vi "Waveplate control panel.vi"(4 "PC WP angle":dbl, 5 "Left or right?":dbl(ring)=80.7 items=["Equal"=58.2, "Right"=35.7, "Left"=80.7], 6 "Pump WP angle":dbl, 7 "Waveplate or Pockels cell?":dbl(ring)=55.98 items=["Waveplate"=71.5, "Pockels cell"=26.5], 8 "L/R WP angle":dbl, 9 "Manual?":bool, 10 "Move waveplates":bool, 11 "Home Button":bool) -> (2 "VISA handle out":refnum<visa-resource-name>, 3 "Final positions":dbl[](array[numeric]))   [LabVIEW 2013]
doc: "Demonstrates the fundamentals of the State Machine design pattern in LabVIEW. A state machine, in its simplest form, is a case structure within a while loop, with a state enum wired to a shift register on the loop to define the execution of different cases (or \"states\") of the case structure on different iterations of the loop."
uses:
  Source/State Machine Fundamentals - State Enum.ctl
panel:
  in  "Axis 3\n(Pump)":bool=TRUE
  in  "Axis 2\n(WP/PC)":bool=TRUE
  in  "Axis 1\n(L/R)":bool=TRUE
  in  "Serial port":u8=3
  out "Moving":bool
  out "Initializing":bool
  out "Error out":errorcluster
  out "Moving axis":i32
  in  "Error in":errorcluster
  in  "Stop":bool
  # "Instructions: Start VI. All three SMC100 motion controllers will automatically initialize; this will\ntake several seconds for each and requires homing the stages. Choose waveplate/Pockels cell\nand left/right, OR turn on Manual and set desired angles for each stage. The pump waveplate\nalways uses its manual value. Press Move Waveplates to initiate motion. If any stage gives a \n\"Controller is not in the ready state\" error, it may be necessary to re-initialize by pressing Initialize."
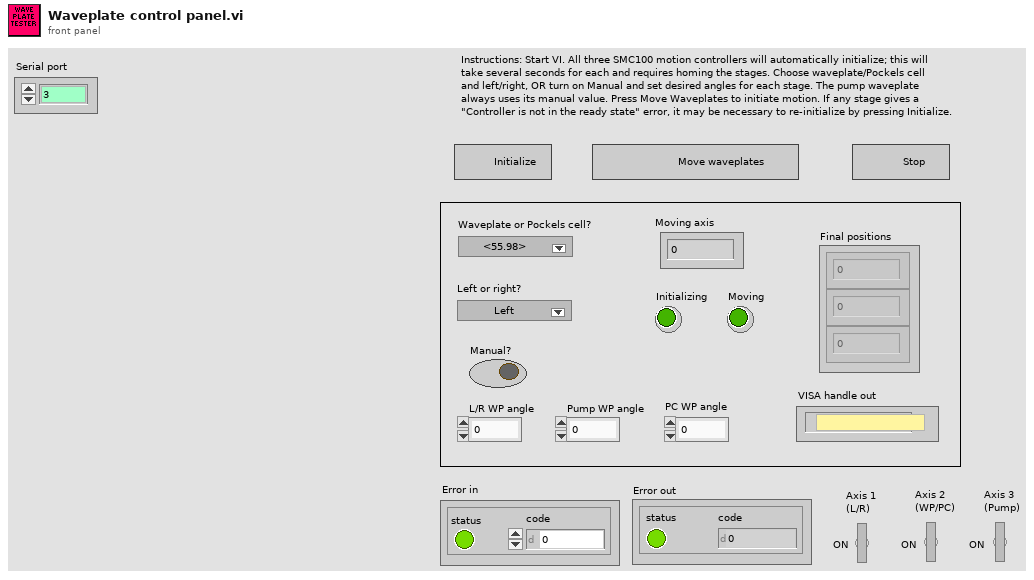
[diagram p1: front panel]
types:
  T1 = typedef "State Machine Fundamentals - State Enum.ctl" = enum16{"Initialize", "Wait for go", "Move", "Stop"}
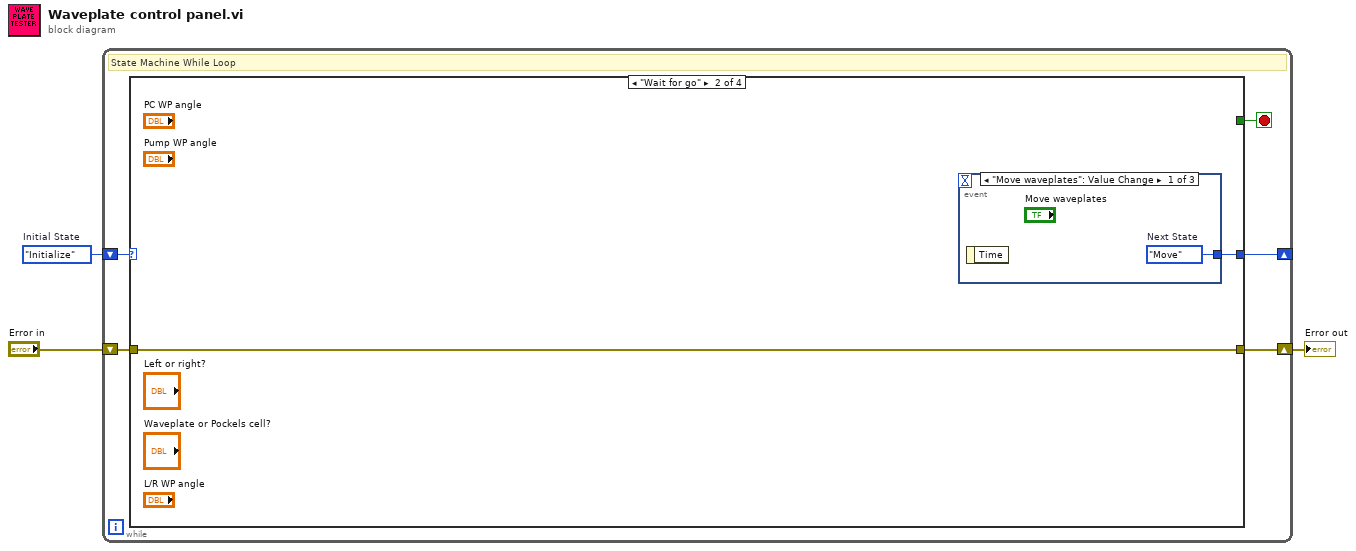
[diagram p0: block diagram]
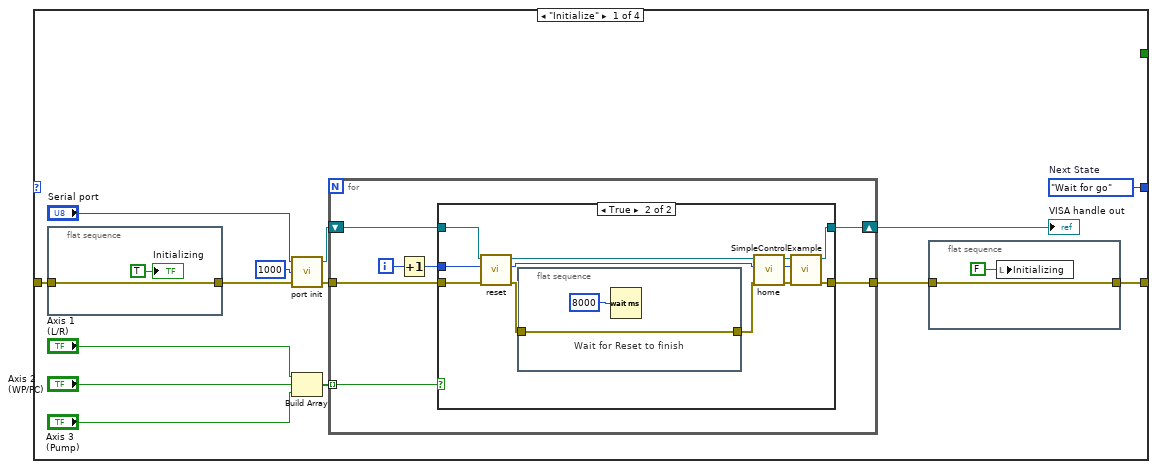
[diagram p2: hidden frame]
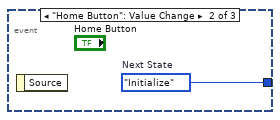
[diagram p4: hidden frame]
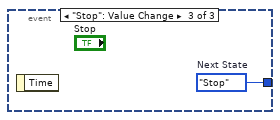
[diagram p5: hidden frame]
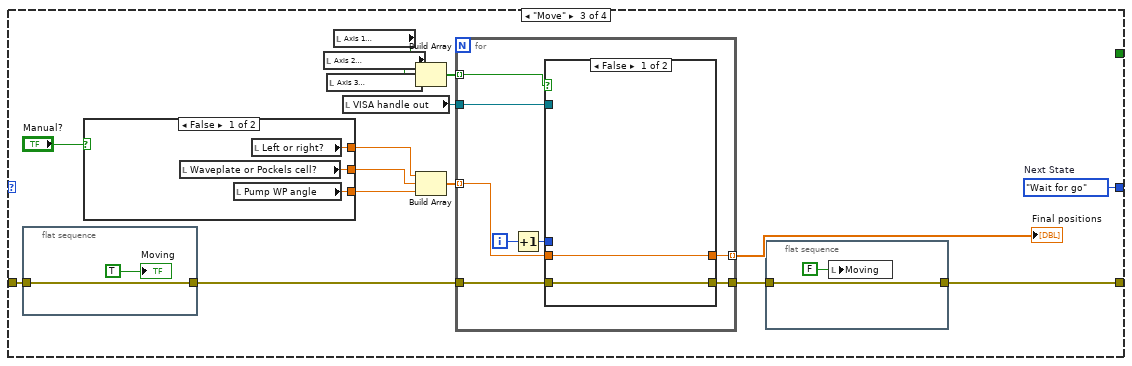
[diagram p6: hidden frame]
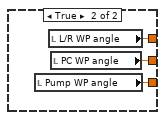
[diagram p7: hidden frame]
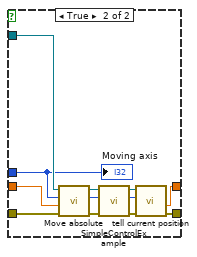
[diagram p8: hidden frame]
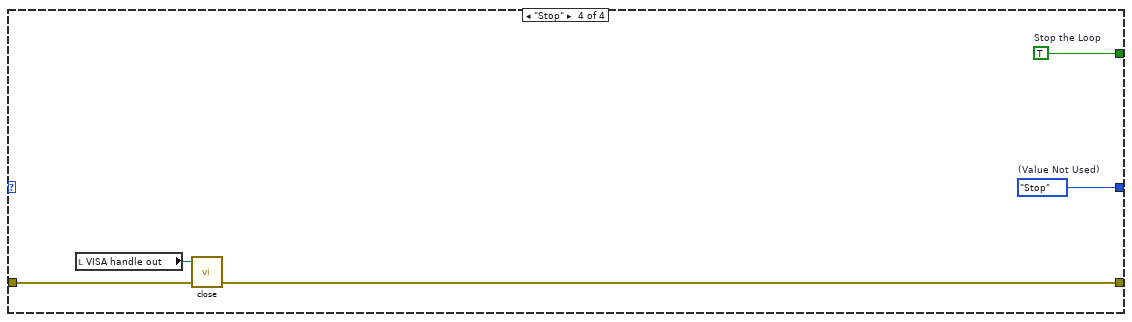
[diagram p9: hidden frame]
diagram:
  w3 = State_Machine_Fundamentals_-_State_Enum."Initialize"  # Initial State
  n1 = while {
    shift-right: [w7] -> _
    shift-left: w3 -> [w8]
    shift-right: [w4] -> w1
    shift-left: "Error in" -> [w5]
    stop <- w6 stop-if-true
    # "State Machine While Loop"
    n2 = case "State Machine Case Structure" shown="\"Wait for go\"" w8 {
      tunnel: [w22 w51 w69 w107] -> w7
      tunnel: [_ _ _ w106] -> w6
      tunnel: w5 -> [w21 w50 w64 w105]
      tunnel: [w20 w50 w61 w104] -> w4
      frame "Initialize" {
        w22 = State_Machine_Fundamentals_-_State_Enum."Wait for go"  # Next State
        n3 = flat-sequence {
          tunnel: w21 -> [w49]
          tunnel: [w49] -> w15
          frame #0 {
            "Initializing" <- TRUE ("Initializing")
          }
        }
        n4 = call "port init.vi"("error in"=w15, "Timeout (ms)"=u32 1000 ("Timeout (300 ms)"), "SerialPort"="Serial port") -> ("error out"=w14:errorcluster, "Visa Handle"=w16:refnum<visa-resource-name>)  [unwired: 1 in]
        n5 = Build Array("Axis 1\n(L/R)", "Axis 2\n(WP/PC)", "Axis 3\n(Pump)") -> (w9:bool[])
        n6 = for {
          tunnel: w14 -> [w27]
          shift-right: [w29] -> w19
          shift-left: w16 -> [w28]
          tunnel: [w26] -> w13
          tunnel: w9 -> [w23] mode=indexing
          i -> [w25]
          n7 = Increment(x=w25) -> (x+1=w24:i32)
          n8 = case shown="True" w23 {
            tunnel: [w31 w36] -> w29
            tunnel: w28 -> [w31 w35]
            tunnel: w27 -> [w30 w34]
            tunnel: [w30 w33] -> w26
            tunnel: w24 -> [_ w32]
            frame False {
            }
            frame True {
              n9 = call "reset.vi"("error in"=w34, "Axis in"=w32, "VISA Handle in"=w35) -> ("error out"=w39:errorcluster, "Axis out"=w40:i32, "VISA Handle out"=w37:refnum<visa-resource-name>)  [unwired: 3 in, 1 out]
              n10 = flat-sequence {
                tunnel: [w44] -> w38
                tunnel: w39 -> [w44]
                frame #0 {
                  # "Wait for Reset to finish"
                  n11 = Wait (ms)(milliseconds to wait=u32 8000) -> ()  [unwired: 1 out]
                }
              }
              n12 = call "home.vi"("error in"=w38, "Axis in"=w40, "VISA Handle in"=w37) -> ("error out"=w42:errorcluster, "Axis out"=w41:i32, "VISA Handle out"=w43:refnum<visa-resource-name>)  [unwired: 3 in, 1 out]
              n13 = call "SimpleControlExample.vi"("error in"=w42, "Axis in"=w41, "VISA Handle in"=w43) -> ("error out"=w33:errorcluster, "VISA Handle out"=w36:refnum<visa-resource-name>)  [unwired: 2 in, 3 out]
            }
          }
        }
        "VISA handle out" <- w19
        n14 = flat-sequence {
          tunnel: w13 -> [w47]
          tunnel: [w47] -> w20
          frame #0 {
            n15 = local write "Initializing"(FALSE ("Initializing")) -> ()
          }
        }
      }
      frame "Wait for go" {
        # "Wait for Event - An Event Structure is used to monitor the user interface for events. In each frame of the Event Structure, the next state of the state machine is specified based on which button was pressed."
        n16 = event shown="[0] \"Move waveplates\": Value Change" {
          selector: _ -> [_ _ _]
          dyn-events: _ -> [_ _ _]
          timeout: _ -> [_ _ _]
          tunnel: [w52 w53 w54] -> w51
          event "Move waveplates": Value Change {
            w52 = State_Machine_Fundamentals_-_State_Enum."Move"  # Next State
            n17 = event-data() -> ()  [unwired: 1 in, 1 out]
          }
          event "Home Button": Value Change {
            w53 = State_Machine_Fundamentals_-_State_Enum."Initialize"  # Next State
            n18 = event-data() -> ()  [unwired: 1 in, 1 out]
          }
          event "Stop": Value Change {
            w54 = State_Machine_Fundamentals_-_State_Enum."Stop"  # Next State
            n19 = event-data() -> ()  [unwired: 1 in, 1 out]
          }
        }
      }
      frame "Move" {
        w69 = State_Machine_Fundamentals_-_State_Enum."Wait for go"  # Next State
        # "State 1 - Display a dialog box with a message specific to State 1, then go back to the Wait for Event state."
        n20 = flat-sequence {
          tunnel: w64 -> [w80]
          tunnel: [w80] -> w63
          frame #0 {
            "Moving" <- TRUE ("Moving")
          }
        }
        n21 = case shown="False" "Manual?" {
          tunnel: [w73 w76] -> w67
          tunnel: [w72 w75] -> w66
          tunnel: [w71 w74] -> w59
          frame False {
            n22 = local read "Waveplate or Pockels cell?"() -> (w72:dbl)
            n23 = local read "Pump WP angle"() -> (w71:dbl)
            n24 = local read "Left or right?"() -> (w73:dbl)
          }
          frame True {
            n25 = local read "Pump WP angle"() -> (w74:dbl)
            n26 = local read "L/R WP angle"() -> (w76:dbl)
            n27 = local read "PC WP angle"() -> (w75:dbl)
          }
        }
        n28 = local read "Axis 2\n(WP/PC)"() -> (w57:bool)
        n29 = local read "Axis 3\n(Pump)"() -> (w56:bool)
        n30 = local read "Axis 1\n(L/R)"() -> (w58:bool)
        n31 = local read "VISA handle out"() -> (w65:refnum<visa-resource-name>)
        n32 = Build Array(w58, w57, w56) -> (w55:bool[])
        n33 = Build Array(w67, w66, w59) -> (w68:dbl[])
        n34 = for {
          tunnel: [w88] -> w70 mode=indexing
          tunnel: w63 -> [w87]
          tunnel: [w86] -> w62
          tunnel: w68 -> [w85] mode=indexing
          tunnel: w65 -> [w84]
          tunnel: w55 -> [w83] mode=indexing
          i -> [w82]
          n35 = Increment(x=w82) -> (x+1=w81:i32)
          n36 = case shown="False" w83 {
            tunnel: [w89 w102] -> w88
            tunnel: w87 -> [w90 w101]
            tunnel: [w90 w100] -> w86
            tunnel: w85 -> [w89 w99]
            tunnel: w84 -> [_ w98]
            tunnel: w81 -> [_ w91]
            frame False {
            }
            frame True {
              n37 = call "Move absolute.vi"("error in"=w101, "New target position (units)"=w99, "Axis in"=w91, "VISA Handle in"=w98) -> ("error out"=w92:errorcluster, "Axis out"=w93:i32, "VISA Handle out"=w94:refnum<visa-resource-name>)  [unwired: 2 in, 1 out]
              n38 = call "SimpleControlExample.vi"("error in"=w92, "Axis in"=w93, "VISA Handle in"=w94) -> ("error out"=w95:errorcluster, "Axis out"=w96:i32, "VISA Handle out"=w97:refnum<visa-resource-name>)  [unwired: 2 in, 2 out]
              n39 = call "tell current position.vi"("error in"=w95, "Axis in"=w96, "VISA Handle in"=w97) -> ("error out"=w100:errorcluster, "Current position (units)"=w102:dbl)  [unwired: 2 in, 3 out]
              "Moving axis" <- w91
            }
          }
        }
        "Final positions" <- w70
        n40 = flat-sequence {
          tunnel: w62 -> [w77]
          tunnel: [w77] -> w61
          frame #0 {
            n41 = local write "Moving"(FALSE ("Moving")) -> ()
          }
        }
      }
      frame "Stop" {
        w106 = TRUE  # Stop the Loop
        w107 = State_Machine_Fundamentals_-_State_Enum."Stop"  # (Value Not Used)
        # "Stop - Stop the VI. This is the only state that specifies a TRUE value for the loop conditional terminal."
        n42 = local read "VISA handle out"() -> (w103:refnum<visa-resource-name>)
        n43 = call "close.vi"("error in"=w105, "VISA Handle in"=w103) -> ("error out"=w104:errorcluster)  [unwired: 3 in]
      }
    }
  }
  "Error out" <- w1
